vi "Log Events.vi"(8 "error in":errorcluster, 10 "Item Names":string[](array[string]), 11 "Event Folder Path":path) -> (0 "error out":errorcluster)   [LabVIEW 2021, in "Game of Life.lvlib"]
doc: "Logs the event record to a CSV file."
uses:
  Game of Life.lvlib
  <vilib>/Utility/file.llb/Write Delimited Spreadsheet (string).vi
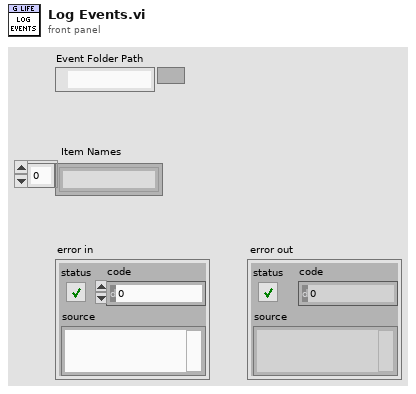
[diagram p1: front panel]
types:
  T1 = enum16{"open", "replace", "create", "open or create", "replace or create", "replace or create with confirmation"}
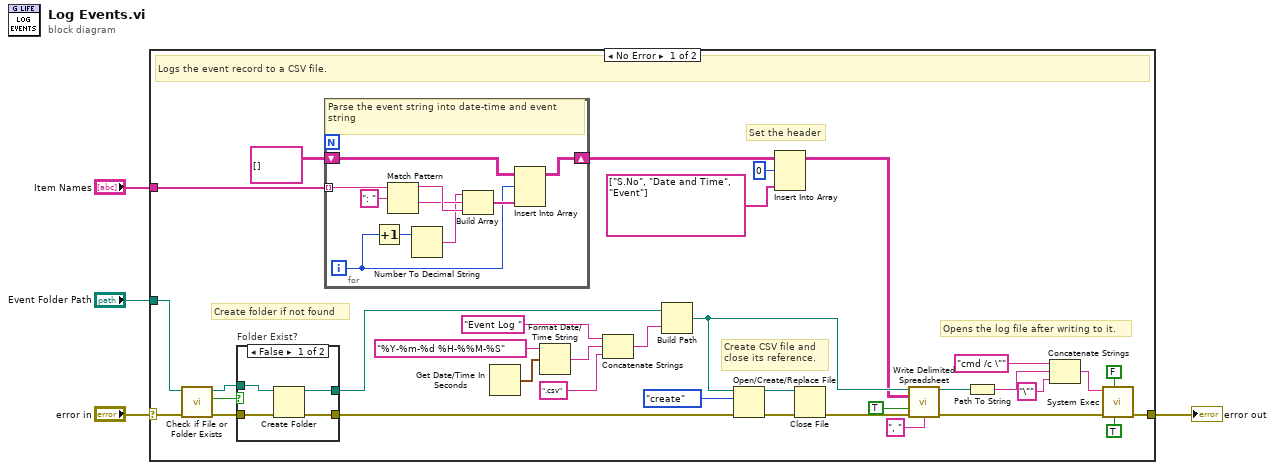
[diagram p0: block diagram]
diagram:
  n1 = case shown="No Error" "error in" {
    selector: "error in" -> [w25 w56]
    tunnel: "Event Folder Path" -> [w26 _]
    tunnel: "Item Names" -> [w34 _]
    tunnel: [w6 w56] -> w1
    frame No Error {
      # "Opens the log file after writing to it."
      # "Create CSV file and \nclose its reference."
      # "Create folder if not found"
      # "Set the header"
      # "Logs the event record to a CSV file."
      n2 = call <vilib>:"Check if File or Folder Exists.vi"("error in (no error)"=w25, "path"=w26) -> ("error out"=w23:errorcluster, "file or folder exists?"=w24:bool, "dup path"=w22:path)  [unwired: 7 in]
      n3 = case "Folder Exist?" shown="False" w24 {
        tunnel: w23 -> [w43 w45]
        tunnel: [w42 w45] -> w20
        tunnel: w22 -> [w41 w44]
        tunnel: [w40 w44] -> w21
        frame False {
          n4 = Create Folder(path (use dialog)=w41, error in=w43) -> (created path=w40:path, error out=w42:errorcluster)  [unwired: 1 in, 1 out]
        }
        frame True {
        }
      }
      n5 = for {
        tunnel: w34 -> [w55] mode=indexing
        shift-right: [w49] -> w17
        shift-left: string[][] [] ("Item Names") -> [w50]
        i -> [w48]
        # "Parse the event string into date-time and event string"
        n6 = Increment(x=w48) -> (x+1=w47:i32)
        n7 = Match Pattern(string=w55, regular expression=": ") -> (before substring=w53:string, after substring=w52:string)  [unwired: 1 in, 2 out]
        n8 = Number To Decimal String(number=w47) -> (decimal integer string=w46:string)  [unwired: 1 in]
        n9 = Build Array(w46, w52, w53) -> (w51:string[])
        n10 = Insert Into Array(array=w50, index (row)=w48, new element=w51) -> (w49:string[][])  [unwired: 1 in]
      }
      n11 = Get Date/Time In Seconds() -> (seconds since 1Jan1904=w36:timestamp)
      n12 = Format Date/Time String(time format string (%c)="%Y-%m-%d %H-%%M-%S", seconds (now)=w36) -> (date/time string=w38:string)  [unwired: 1 in]
      n13 = Concatenate Strings("Event Log " ("string"), w38, ".csv" ("string")) -> (w37:string)
      n14 = Build Path(base path=w21, name or relative path=w37) -> (appended path=w29:path)
      n15 = Open/Create/Replace File(file path (use dialog)=w29, error in=w20, operation (0:open)=T1."create") -> (refnum out=w30:refnum<file>, error out=w32:errorcluster)  [unwired: 3 in, 1 out]
      n16 = Insert Into Array(array=w17, index (row)=0, new element=string[] ["S.No", "Date and Time", "Event"] ("new element/subarray")) -> (w16:string[][])  [unwired: 1 in]
      n17 = Close File(refnum=w30, error in=w32) -> (error out=w31:errorcluster)  [unwired: 1 out]
      n18 = call-poly <vilib>:"Write Delimited Spreadsheet.vi"("file path (dialog if empty)"=w29, "2D data"=w16, "append to file? (new file:F)"=TRUE, "error in (no error)"=w31, "delimiter (\\t)"=", " ("delimiter (\\t)")) -> ("new file path (Not A Path if cancelled)"=w5:path, "error out"=w7:errorcluster)  [unwired: 9 in]
      n19 = Path To String(path=w5) -> (string=w12:string)
      n20 = Concatenate Strings("cmd /c \"" ("string"), w12, "\"" ("string")) -> (w10:string)
      n21 = call <vilib>:"System Exec.vi"("run minimized? (F)"=TRUE, "wait until completion? (T)"=FALSE, "error in (no error)"=w7, "command line"=w10) -> ("error out"=w6:errorcluster)  [unwired: 4 in, 3 out]
    }
    frame Error {
    }
  }
  "error out" <- w1
